vi "Image_To_Intensity.vi"(1 "image":T1={"image type"=0, "image depth"=1, "image"=[0, 0, 63, 255, 0, 0, 0, 0, 0, 0, 63, 255, 0, 0, 0, 0, 0, 0, 63, 255, 0, 0, 0, 0, 0, 0, 63, 255, 0, 0, 0, 0, 0, 0, 63, 255, 0, 0, 0, 0, 0, 0, 63, 255, 0, 0, 0, 0, 0, 15, 255, 255, 252, 0, 0, 0, 0, 15, 255, 255, 252, 0, 0, 0, 0, 15, 255, 255, 252, 0, 0, 0, 0, 15, 255, 255, 252, 0, 0, 0, 0, 15, 255, 255, 252, 0, 0, 0, 0, 15, 255, 255, 252, 0, 0, 0, 3, 255, 255, 255, 255, 240, 0, 0, 3, 255, 255, 255, 255, 240, 0, 0, 3, 255, 255, 255, 255, 240, 0, 0, 3, 255, 255, 255, 255, 240, 0, 0, 3, 255, 255, 255, 255, 240, 0, 0, 3, 255, 255, 255, 255, 240, 0, 0, 255, 255, 255, 255, 255, 255, 192, 0, 255, 248, 63, 255, 7, 255, 192, 0, 255, 248, 63, 255, 7, 255, 192, 0, 255, 248, 63, 255, 7, 255, 192, 0, 255, 248, 63, 255, 7, 255, 192, 0, 255, 248, 63, 255, 7, 255, 192, 0, 255, 248, 63, 255, 7, 255, 192, 0, 255, 255, 255, 255, 255, 255, 192, 0, 255, 255, 255, 255, 255, 255, 192, 0, 255, 255, 255, 255, 255, 255, 192, 0, 255, 255, 255, 255, 255, 255, 192, 0, 255, 255, 255, 255, 255, 255, 192, 0, 255, 255, 255, 255, 255, 255, 192, 0, 255, 255, 255, 255, 255, 255, 192, 0, 0, 15, 224, 1, 252, 0, 0, 0, 0, 15, 224, 1, 252, 0, 0, 0, 0, 15, 224, 1, 252, 0, 0, 0, 0, 15, 224, 1, 252, 0, 0, 0, 0, 15, 224, 1, 252, 0, 0, 0, 3, 255, 255, 255, 255, 240, 0, 0, 3, 248, 63, 255, 7, 240, 0, 0, 3, 248, 63, 255, 7, 240, 0, 0, 3, 248, 63, 255, 7, 240, 0, 0, 3, 248, 63, 255, 7, 240, 0, 0, 3, 248, 63, 255, 7, 240, 0, 0, 255, 255, 255, 255, 255, 255, 192, 0, 254, 15, 224, 1, 252, 31, 192, 0, 254, 15, 224, 1, 252, 31, 192, 0, 254, 15, 224, 1, 252, 31, 192, 0, 254, 15, 224, 1, 252, 31, 192, 0, 254, 15, 224, 1, 252, 31, 192, 0, 254, 15, 224, 1, 252, 31, 192, 0], "mask"=[], "colors"=[0, 16777215], "Rectangle"={"left"=0, "top"=0, "right"=50, "bottom"=50}}) -> (0 "Intensity Graph":u8[][](graph))   [LabVIEW 2022 SP3]
uses:
  <vilib>/picture/picture.llb/imagedata.ctl
panel:
  out "Numeric":i32
  out "Array":u32[](array[numeric])
  out "size(s)":i32[](array[numeric])
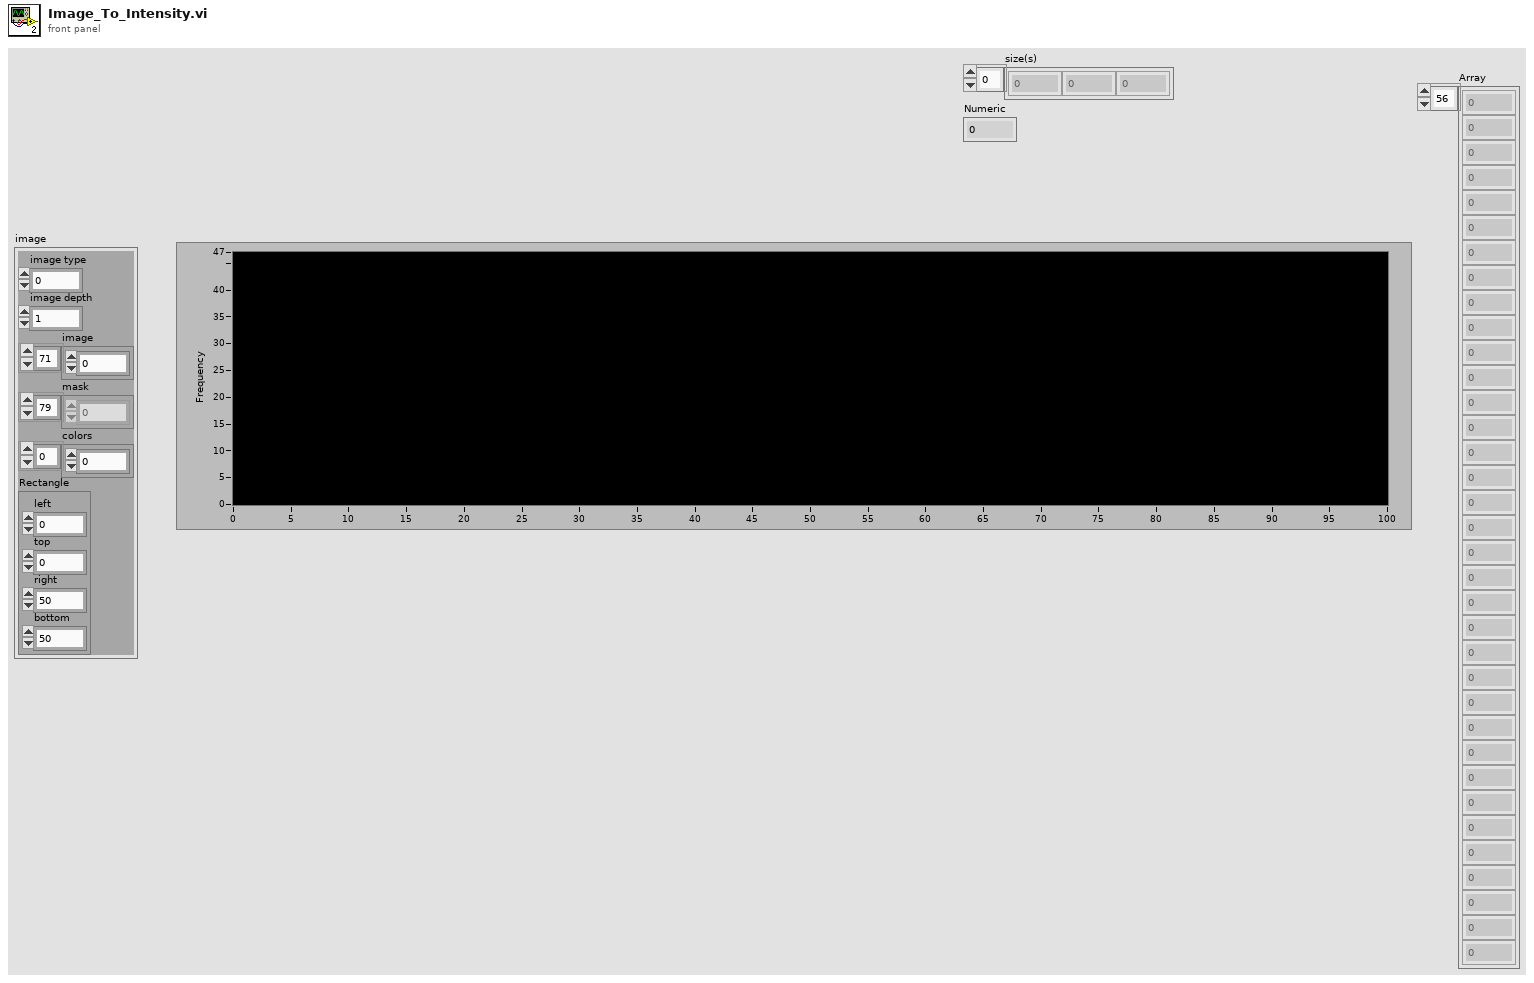
[diagram p1: front panel]
types:
  T1 = typedef "imagedata.ctl" = cluster{"image type":i32, "image depth":i32, "image":u8[], "mask":u8[], "colors":u32[], "Rectangle":cluster{"left":i16, "top":i16, "right":i16, "bottom":i16}}
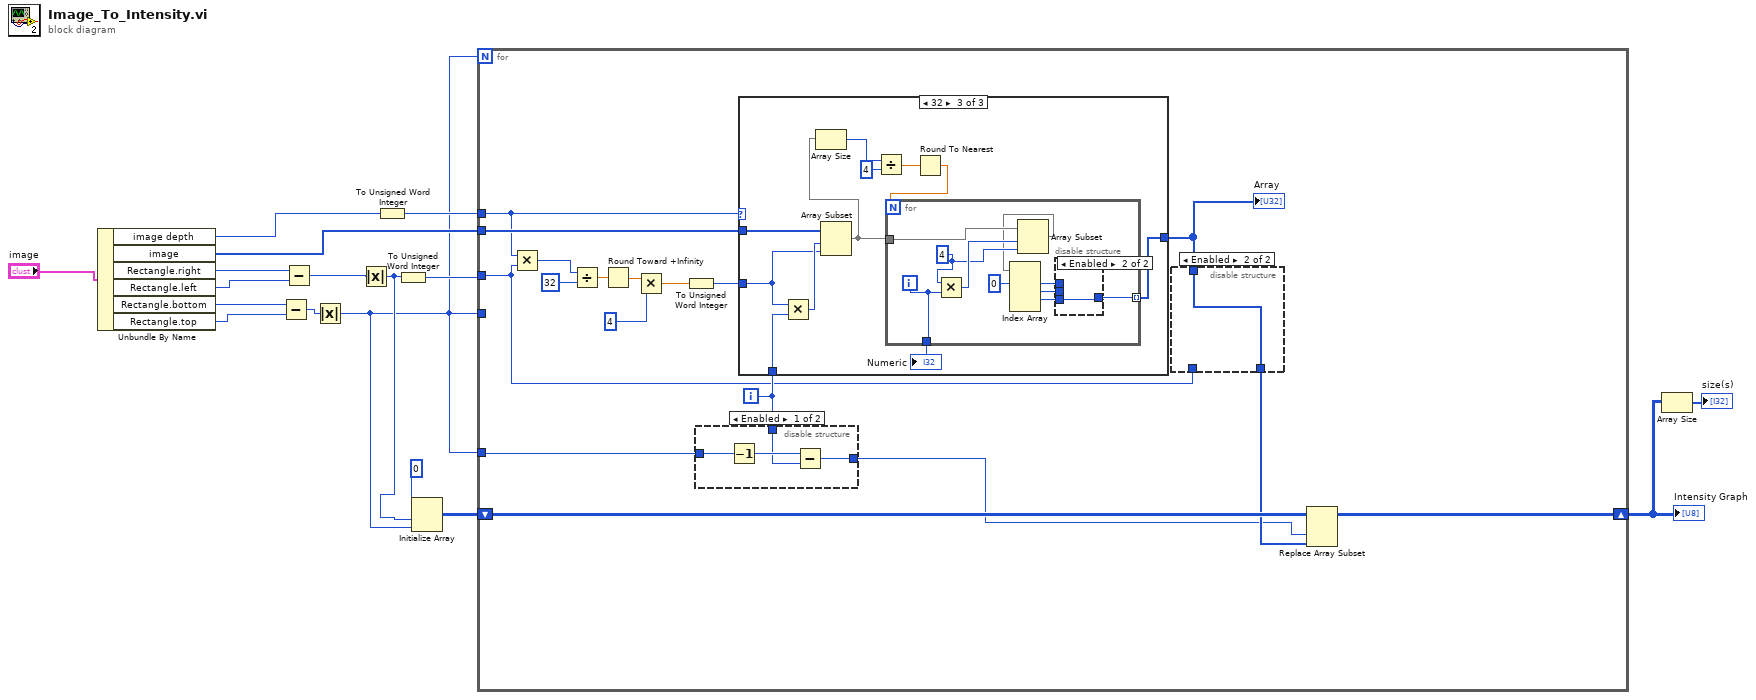
[diagram p0: block diagram]
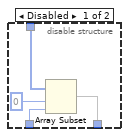
[diagram p2: hidden frame]
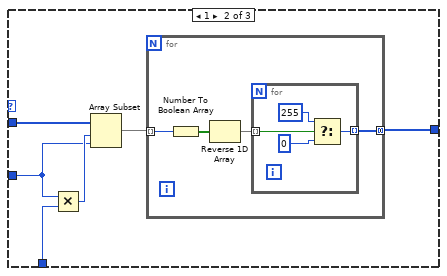
[diagram p5: hidden frame]
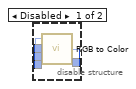
[diagram p6: hidden frame]
diagram:
  n1 = Unbundle By Name("image") -> ("image depth"=w10:i32, "image"=w15:u8[], "Rectangle.right"=w12:i16, "Rectangle.left"=w11:i16, "Rectangle.bottom"=w14:i16, "Rectangle.top"=w13:i16)
  n2 = Subtract(x=w14, y=w13) -> (x-y=w5:i16)
  n3 = Subtract(x=w12, y=w11) -> (x-y=w7:i16)
  n4 = Absolute Value(x=w5) -> (abs(x)=w4:i16)
  n5 = Absolute Value(x=w7) -> (abs(x)=w6:i16)
  n6 = To Unsigned Word Integer(number=w10) -> (unsigned 16bit integer=w9:u16)
  n7 = To Unsigned Word Integer(number=w6) -> (unsigned 16bit integer=w8:u16)
  n8 = Initialize Array(u8 0, w6, w4) -> (w16:u8[][])
  n9 = for {
    N: w4 -> [_]
    shift-right: [w19] -> w2
    shift-left: w16 -> [w23]
    tunnel: w15 -> [w34]
    tunnel: w4 -> [w33]
    tunnel: w8 -> [w22]
    tunnel: w4 -> [_]
    tunnel: w9 -> [w31]
    i -> [w32]
    n10 = Multiply(x=w31, y=w22) -> (x*y=w30:u16)
    n11 = Divide(x=w30, y=32) -> (x/y=w28:dbl)
    n12 = Round Toward +Infinity(x=w28) -> (ceil(x): smallest int >= x=w27:dbl)
    n13 = Multiply(x=w27, y=u16 4) -> (x*y=w24:dbl)
    n14 = To Unsigned Word Integer(number=w24) -> (unsigned 16bit integer=w25:u16)
    n15 = disable-structure shown="Enabled" {
      disable-tunnel: w33 -> [w43 _]
      disable-tunnel: w32 -> [w41 w44]
      disable-tunnel: [w40 w44] -> w18
      frame Enabled {
        n16 = Decrement(x=w43) -> (x-1=w42:i16)
        n17 = Subtract(x=w42, y=w41) -> (x-y=w40:i32)
      }
      frame Disabled {
      }
    }
    n18 = case shown="32" w31 {
      tunnel: w34 -> [_ w50 w69]
      tunnel: [_ w47 w60] -> w20
      tunnel: w32 -> [_ w46 w67]
      tunnel: w25 -> [_ w45 w66]
      frame Default {
      }
      frame 1 {
        n19 = Multiply(x=w45, y=w46) -> (x*y=w49:i32)
        n20 = Array Subset(array=w50, index=w49, length=w45) -> (w48:u8[])
        n21 = for {
          tunnel: w48 -> [w51] mode=indexing
          tunnel: [w54] -> w47 mode=concatenating
          n22 = Number To Boolean Array(number=w51) -> (Boolean array=w53:bool[])
          n23 = Reverse 1D Array(array=w53) -> (reversed array=w52:bool[])
          n24 = for {
            tunnel: w52 -> [w58] mode=indexing
            tunnel: [w55] -> w54 mode=indexing
            n25 = Select(t=u8 255, s=w58, f=u8 0) -> (s? t:f=w55:u8)
          }
        }
      }
      frame 32 {
        n26 = Multiply(x=w66, y=w67) -> (x*y=w68:i32)
        n27 = Array Subset(array=w69, index=w68, length=w66) -> (w65:u8[])
        n28 = Array Size(array=w65) -> (size(s)=w64:i32)
        n29 = Divide(x=w64, y=4) -> (x/y=w62:dbl)
        n30 = Round To Nearest(number=w62) -> (nearest integer value=w61:dbl)
        n31 = for {
          N: w61 -> [_]
          tunnel: [w75] -> w60 mode=indexing
          tunnel: [w74] -> w59
          tunnel: w65 -> [w73]
          i -> [w74]
          w71 = 4 ("length")
          n32 = Multiply(x=w71, y=w74) -> (x*y=w72:i32)
          n33 = Array Subset(array=w73, index=w72, length=w71) -> (w70:u8[])
          n34 = Index Array(array=w70, index #1=0 ("index")) -> (element #1=w78:u8, element #2=w77:u8, element #3=w76:u8)  [unwired: 3 in, 1 out]
          n35 = disable-structure shown="Enabled" {
            disable-tunnel: w78 -> [w83 _]
            disable-tunnel: w77 -> [w82 _]
            disable-tunnel: w76 -> [w81 w84]
            disable-tunnel: [w80 w84] -> w75
            frame Disabled {
              n36 = call <vilib>:"RGB to Color.vi"("B"=w81, "G"=w82, "R"=w83) -> ("Color"=w80:u32)
            }
            frame Enabled {
            }
          }
        }
        "Numeric" <- w59
      }
    }
    "Array" <- w20
    n37 = disable-structure shown="Enabled" {
      disable-tunnel: w22 -> [w37 _]
      disable-tunnel: [w36 w39] -> w21
      disable-tunnel: w20 -> [w35 w39]
      frame Disabled {
        n38 = Array Subset(array=w35, index=0, length=w37) -> (w36:u8[])
      }
      frame Enabled {
      }
    }
    n39 = Replace Array Subset(array=w23, new element=w21, index (col)=w18) -> (w19:u8[][])  [unwired: 1 in]
  }
  "Intensity Graph" <- w2
  n40 = Array Size(array=w2) -> (size(s)=→"size(s)":i32[])
